vi "ReadSeqFromXMLFile.vi"(8 "error in (no error)":errorcluster, 11 "Sequence in":refnum<class "Sequence.lvclass">) -> (0 "error out":errorcluster, 1 "TestSequence":T1[](array[typedef]), 2 "Valid Seq":bool, 3 "Sequence out":refnum<class "Sequence.lvclass">, 4 "Motion":bool)   [LabVIEW 2019]
doc: "Read test sequence from persistant file on disk. should be the last sequence edited."
uses:
  Sequence.lvclass
  SequenceSubvis/RF Direction.ctl
  SequenceSubvis/PolarizationSelect.ctl
  SequenceSubvis/TestStepTypes.ctl
  SequenceSubvis/TestStep-StepType.ctl
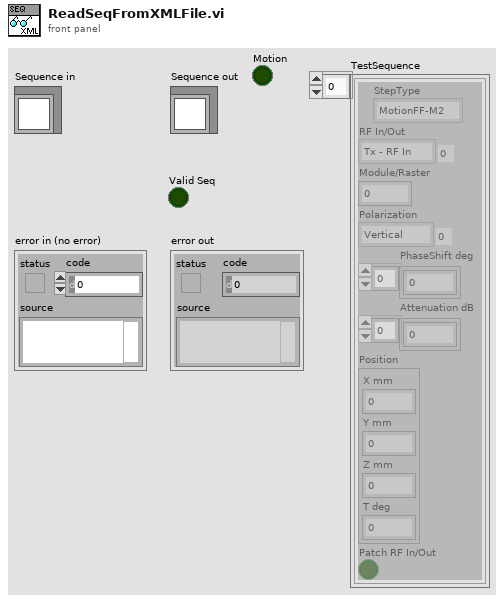
[diagram p1: front panel]
types:
  T1 = typedef "TestStep-StepType.ctl" = cluster{"StepType":T2, "RF In/Out":T3, "Module/Raster":i32, "Polarization":T4, "PhaseShift deg":dbl[], "Attenuation dB":dbl[], "Position":cluster{"X mm":dbl, "Y mm":dbl, "Z mm":dbl, "T deg":dbl}, "Patch RF In/Out":bool}
  T2 = typedef "TestStepTypes.ctl" = enum16{"MotionFF-M2", "Motion", "SweepTest", "RasterTest", "Finish", "64ModuleCfg"}
  T3 = typedef "RF Direction.ctl" = enum16{"Tx - RF In", "Rx - RF Out"}
  T4 = typedef "PolarizationSelect.ctl" = enum16{"Vertical", "Horizontal"}
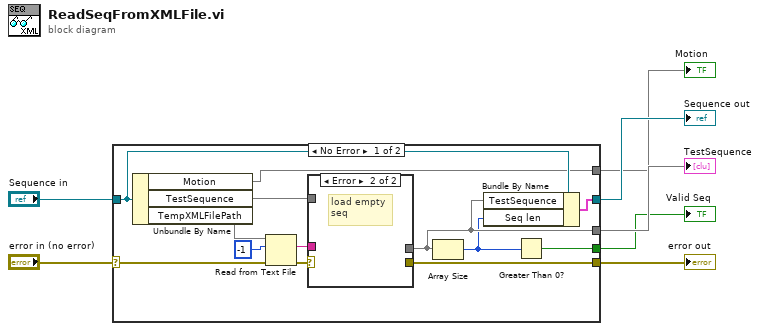
[diagram p0: block diagram]
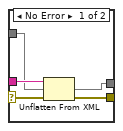
[diagram p2: hidden frame]
diagram:
  n1 = case shown="No Error" "error in (no error)" {
    selector: "error in (no error)" -> [w14 w27]
    tunnel: [w13 w27] -> w6
    tunnel: [w16 w26] -> w4
    tunnel: "Sequence in" -> [w17 w26]
    tunnel: [w11 _] -> w3
    tunnel: [w10 _] -> w2
    tunnel: [w8 _] -> w1
    frame No Error {
      n2 = Unbundle By Name(w17) -> ("Motion"=w8, "TestSequence"=w18, "TempXMLFilePath"=w19)
      n3 = Read from Text File(file (use dialog)=w19, count=-1, error in=w14) -> (text=w20:string, error out=w12:errorcluster)  [unwired: 1 in, 2 out]
      n4 = case shown="Error" w12 {
        selector: w12 -> [w21 _]
        tunnel: w20 -> [w25 _]
        tunnel: w18 -> [w24 _]
        tunnel: [w23 _] -> w11
        tunnel: [w22 _] -> w13
        frame No Error {
          n5 = Unflatten From XML(xml string=w25, type=w24, error in (no error)=w21) -> (value=w23, error out=w22:errorcluster)
        }
        frame Error {
          # "load empty\nseq"
        }
      }
      n6 = Array Size(array=w11) -> (size(s)=w9:i32)
      n7 = Bundle By Name(cluster=w17, "TestSequence"=w11, "Seq len"=w9) -> (w16:cluster{})
      n8 = Greater Than 0?(x=w9) -> (x > 0?=w10:bool)
    }
    frame Error {
    }
  }
  "error out" <- w6
  "Sequence out" <- w4
  "TestSequence" <- w3
  "Valid Seq" <- w2
  "Motion" <- w1
